vi "ValveGUI Main.vi"   [LabVIEW 2020, in "VolatusScratch.lvlib"]
uses:
  VolatusScratch.lvlib
  Volatus/Volatus Core/Volatus Core.lvclass
  VolatusGUIElements/VolatusGUIElements.lvlib
panel:
  # "ValveGUI\nMain"
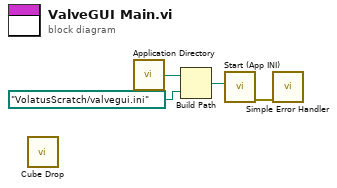
[diagram p0: block diagram]
diagram:
  n1 = call "Cube Drop.vi"() -> ()  [unwired: 12 in]
  n2 = call <vilib>:"Application Directory.vi"() -> ("Application Directory"=w3:path)
  n3 = Build Path(base path=w3, name or relative path=path "VolatusScratch/valvegui.ini") -> (appended path=w1:path)
  n4 = call "Start (App INI).vi"("INI Path (Default)"=w1) -> ("error out"=w4:errorcluster)  [unwired: 9 in, 1 out]
  n5 = call <vilib>:"Simple Error Handler.vi"("error in (no error)"=w4) -> ()  [unwired: 4 in, 5 out]
